vi "get a name.vi"(8 "error constant":errorcluster, 10 "Numeric":i32, 11 "tdms pulse istraction file in":path[](array[path])) -> (0 "error constant 2":errorcluster, 3 "Path":path)   [LabVIEW 2021]
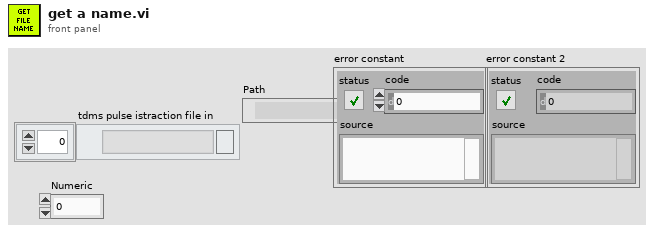
[diagram p1: front panel]
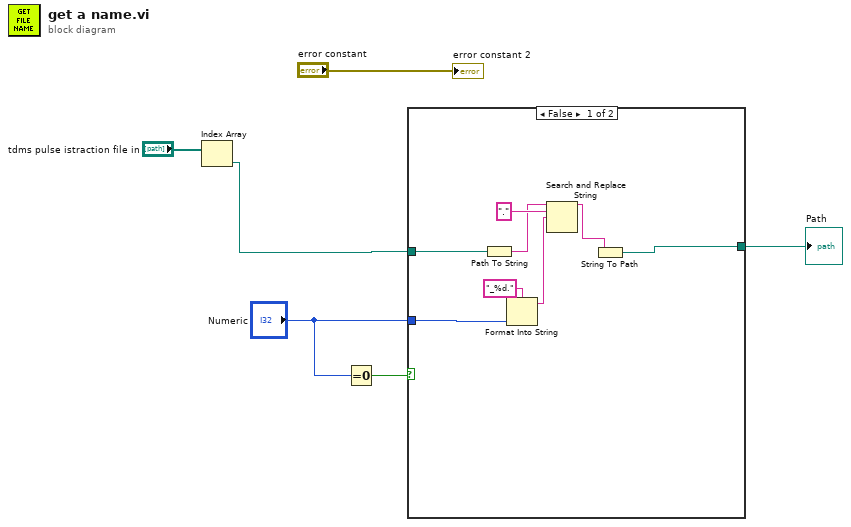
[diagram p0: block diagram]
diagram:
  n1 = Index Array(array="tdms pulse istraction file in") -> (element=w1:path)  [unwired: 1 in]
  n2 = Equal To 0?(x="Numeric") -> (x = 0?=w4:bool)
  n3 = case shown="False" w4 {
    tunnel: [w14 w15] -> w6
    tunnel: w1 -> [w8 w15]
    tunnel: "Numeric" -> [w7 _]
    frame False {
      n4 = Path To String(path=w8) -> (string=w9:string)
      n5 = Format Into String(format string="_%d.", w7) -> (resulting string=w12:string)  [unwired: 2 in, 1 out]
      n6 = Search and Replace String(input string=w9, search string=".", replace string=w12) -> (result string=w10:string)  [unwired: 5 in, 3 out]
      n7 = String To Path(string=w10) -> (path=w14:path)
    }
    frame True {
    }
  }
  "Path" <- w6
  "error constant 2" <- "error constant"
